vi "send_MCUSupportStatus.vi"(4 "Counter":i32, 5 "200/freq":i32=20, 6 "Active":bool, 7 "CAN ID":u32=800 format="%x", 8 "Message":cluster{"SC endline [V]":u8} {"SC endline [V]" scale=0.0..30.0}, 11 "CAN frame":T1[](array[typedef]) {"Data" format="%.0x"; "ArbitrationId" format="%.0x"; "Timestamp" format="%<%I:%M:%S%3u %p\n%m/%d/%Y>T"}) -> (3 "CAN frame out":T1[](array[typedef]) {"Data" format="%.0x"; "ArbitrationId" format="%.0x"; "Timestamp" format="%<%I:%M:%S%3u %p\n%m/%d/%Y>T"})   [LabVIEW 2017]
uses:
  <vilib>/nican/nican.llb/CanFrameTimed.ctl
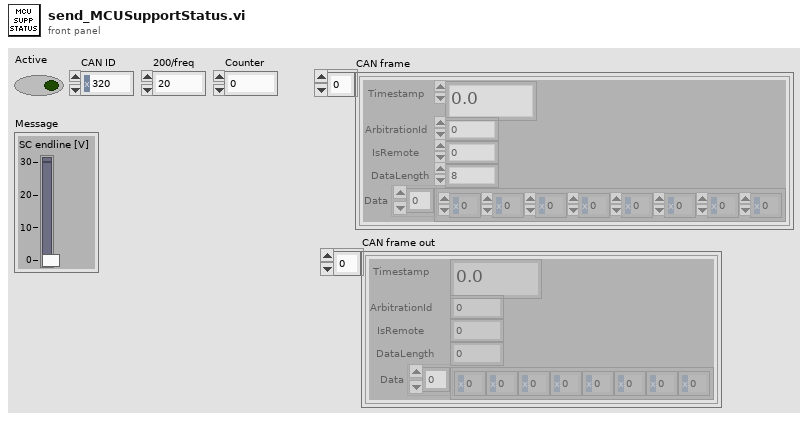
[diagram p1: front panel]
types:
  T1 = typedef "CanFrameTimed.ctl" = cluster{"Timestamp":dbl, "ArbitrationId":u32, "IsRemote":u8, "DataLength":u8, "Data":u8[]}
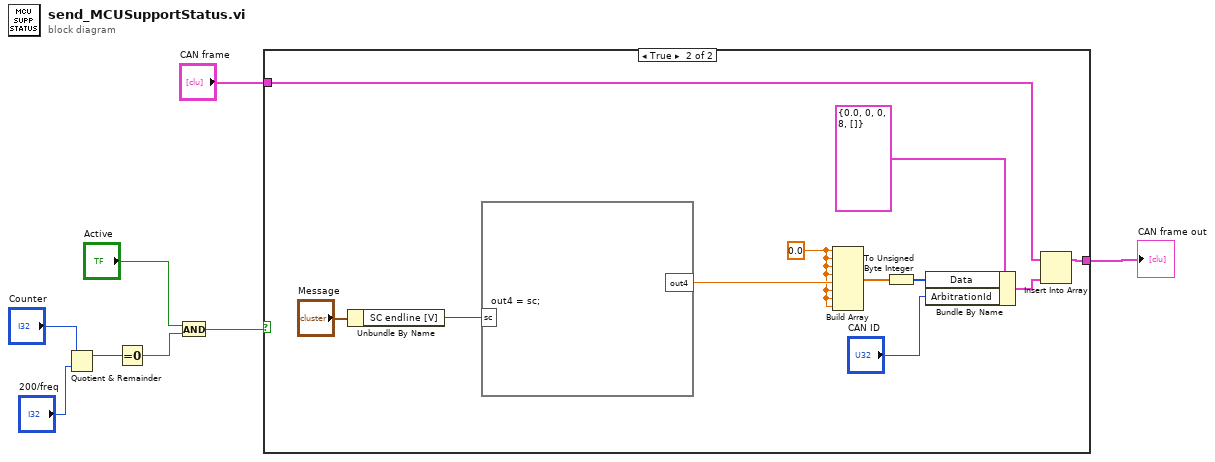
[diagram p0: block diagram]
diagram:
  n1 = Quotient & Remainder(x="Counter", y="200/freq") -> (x-y*floor(x/y)=w5:i32)  [unwired: 1 out]
  n2 = Equal To 0?(x=w5) -> (x = 0?=w3:bool)
  n3 = And(x="Active", y=w3) -> (x .and. y?=w2:bool)
  n4 = case shown="True" w2 {
    tunnel: "CAN frame" -> [w9 w17]
    tunnel: [w9 w15] -> w7
    frame False {
    }
    frame True {
      w10 = 0.0 ("element")
      n5 = Unbundle By Name("Message") -> ("SC endline [V]"=w12:u8)
      n6 = formula code="out4 = sc;"("sc"=w12) -> ("out4"=w11:dbl)
      n7 = Build Array(w10, w10, w10, w10, w11, w10, w10, w10) -> (w20:dbl[])
      n8 = To Unsigned Byte Integer(number=w20) -> (unsigned 8bit integer=w19:u8[])
      n9 = Bundle By Name(cluster=T1 {"Timestamp"=0.0, "ArbitrationId"=0, "IsRemote"=0, "DataLength"=8, "Data"=[]} ("CAN frame"), "Data"=w19, "ArbitrationId"="CAN ID") -> (w16:T1)
      n10 = Insert Into Array(array=w17, new element=w16) -> (w15:T1[])  [unwired: 1 in]
    }
  }
  "CAN frame out" <- w7
